vi "DisablesChannels.vi"(8 "error in":errorcluster, 11 "VISA resource":refnum<visa-resource-name>) -> (0 "error out":errorcluster)   [LabVIEW 2011]
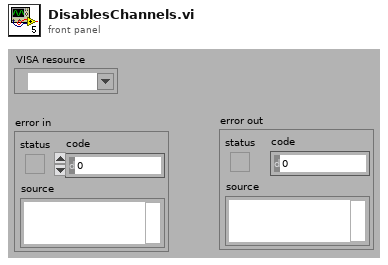
[diagram p1: front panel]
types:
  T1 = enum16{"Initialize", "Write", "Write/Read", "Read", "Clear", "Close"}
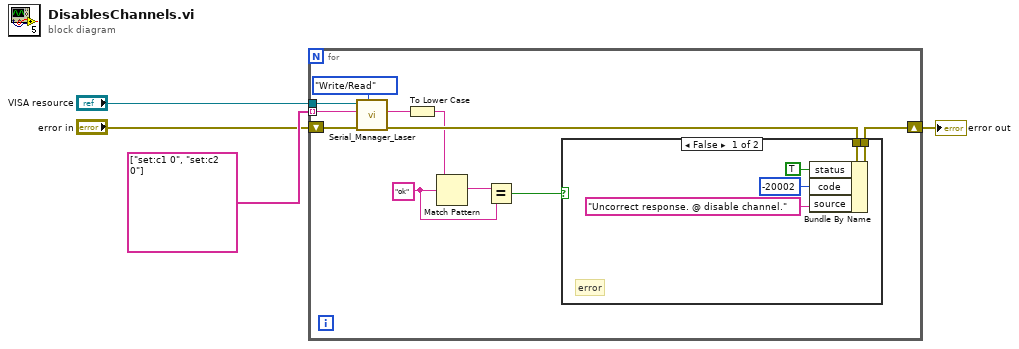
[diagram p0: block diagram]
diagram:
  n1 = for {
    tunnel: "VISA resource" -> [w14]
    tunnel: string[] ["set:c1 0", "set:c2 0"] -> [w11] mode=indexing
    shift-right: [w6] -> w3
    shift-left: "error in" -> [w13]
    w7 = "ok" ("read buffer")
    n2 = call "Serial_Manager_Laser.vi"("Job"=T1."Write/Read", "error in"=w13, "write buffer"=w11, "VISA resource"=w14) -> ("error out"=w12:errorcluster, "read buffer"=w10:string)  [unwired: 6 in]
    n3 = To Lower Case(string=w10) -> (all lower case string=w9:string)
    n4 = Match Pattern(string=w9, regular expression=w7) -> (match substring=w8:string)  [unwired: 1 in, 3 out]
    n5 = Equal?(x=w8, y=w7) -> (x = y?=w5:bool)
    n6 = case shown="False" w5 {
      tunnel: w12 -> [w20 w21]
      tunnel: [w19 w21] -> w6
      frame False {
        # "error"
        n7 = Bundle By Name(cluster=w20, "status"=TRUE, "code"=-20002, "source"="Uncorrect response. @ disable channel.") -> (w19:errorcluster)
      }
      frame True {
      }
    }
  }
  "error out" <- w3
